vi "Main.vi"(8 "error in":errorcluster, 11 "sequenceManagerTest in":refnum<class "sequenceManagerTest.lvclass">) -> (0 "error out":errorcluster, 3 "sequenceManagerTest out":refnum<class "sequenceManagerTest.lvclass">)   [LabVIEW 2023, in "sequenceManagerTest.lvclass"]
doc: "The <b>Queued Message Handler</b> of the Worker that owns this VI."
uses:
  sequenceManagerTest.lvclass
  sequenceManagerTest.lvclass/sequenceManagerTest.ctl
  Initialization Data.ctl
  Response Cases.ctl
  <vilib>/addons/_Workers/Library/Classes/Message Queue/Message Queue.lvclass
  sequenceManagerWorker/sequenceManagerWorker.lvclass
  sequenceManagerWorker/ZE_Easy.Sequencer.lvlibp/Step/Step.lvclass
panel:
  in  "Close Button":bool
  out "Name":string
  out "IsSynchronous":bool
  out "IsParallel":bool
  out "Documentation":string
  in  "Forward Button":bool
  in  "Open Manager":bool
  in  "Path to JSON sequence file":path
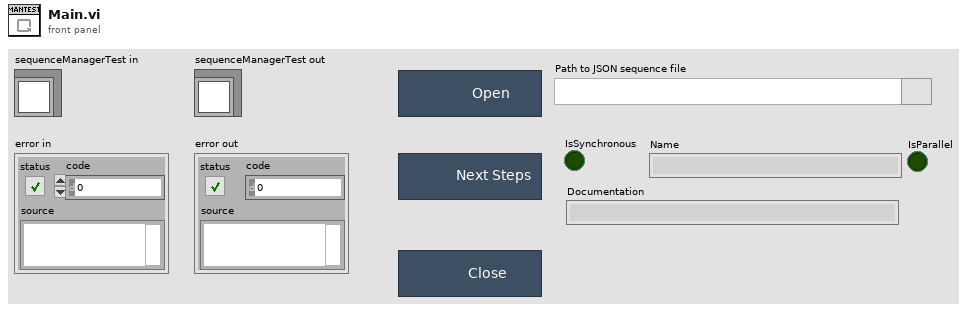
[diagram p1: front panel]
types:
  T1 = typedef "sequenceManagerTest.lvclass/Initialization Data.ctl" = cluster{"Response Cases":T2}
  T2 = typedef "sequenceManagerTest.lvclass/Response Cases.ctl" = cluster{"Placeholder - Can be deleted":string}
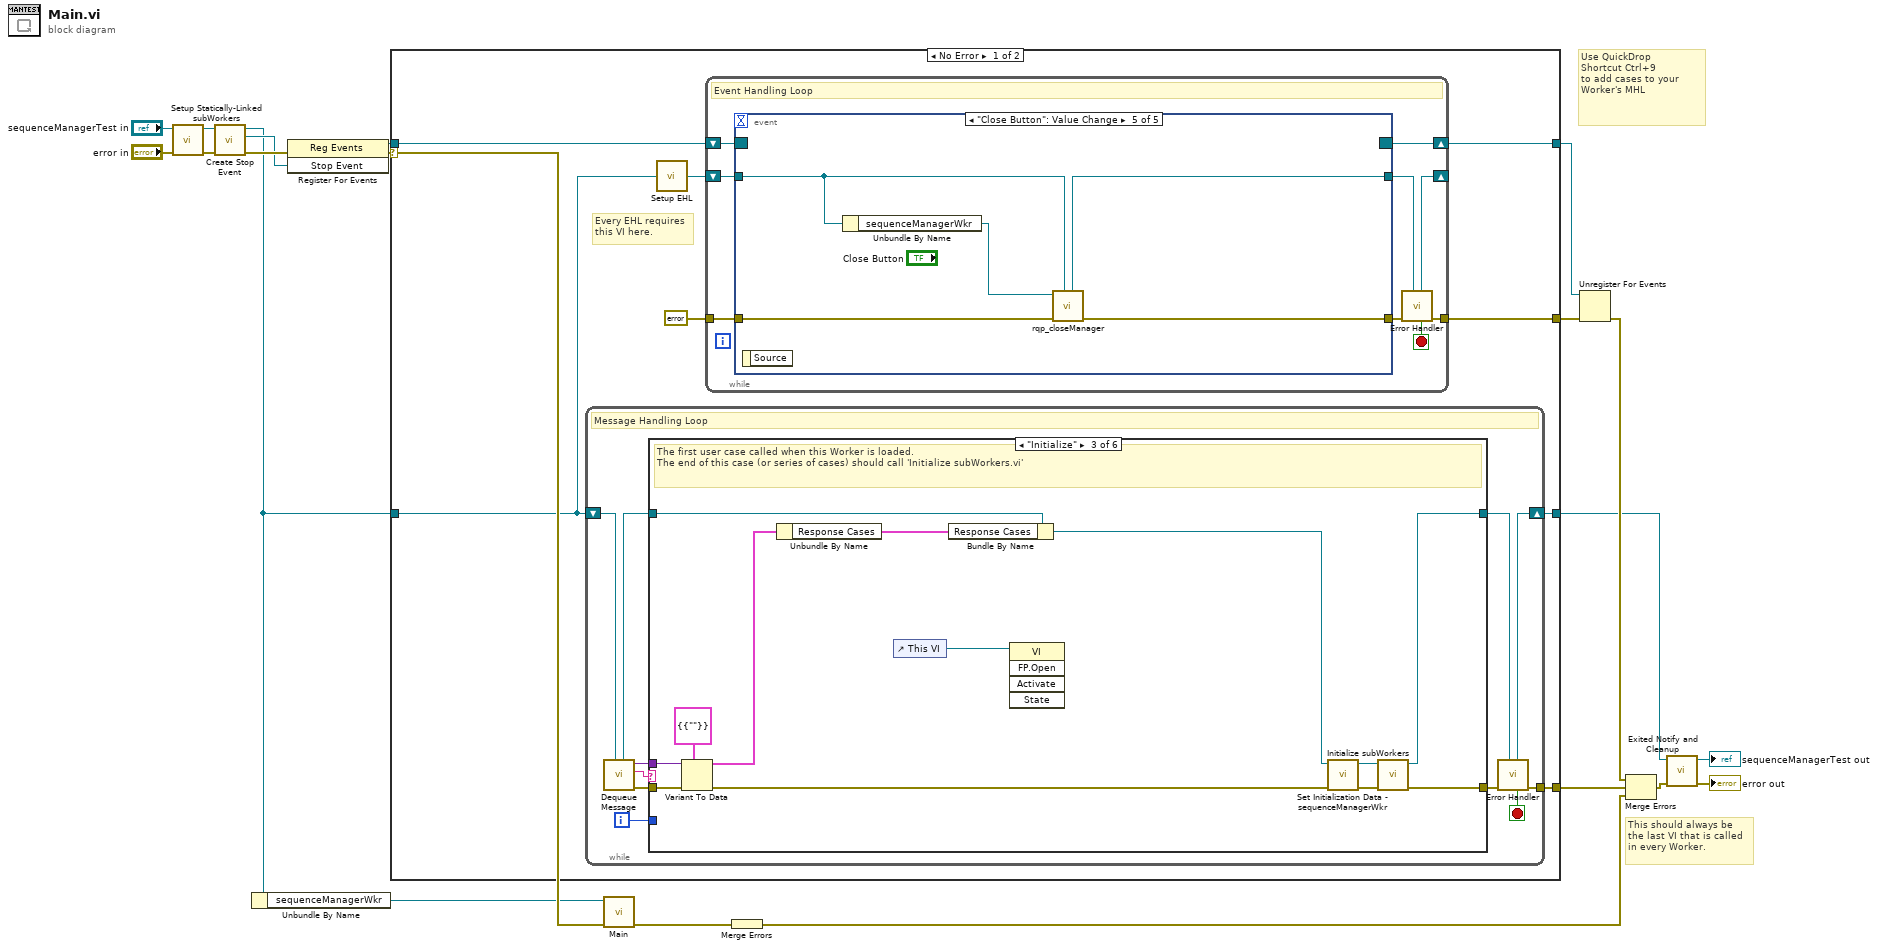
[diagram p0: block diagram]
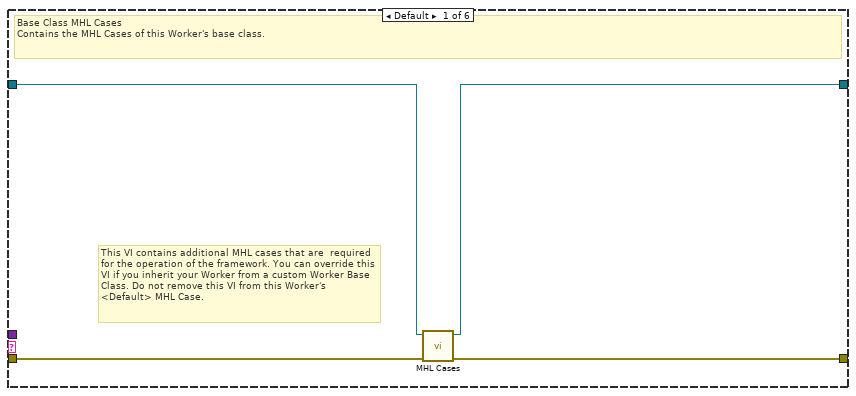
[diagram p2: hidden frame]
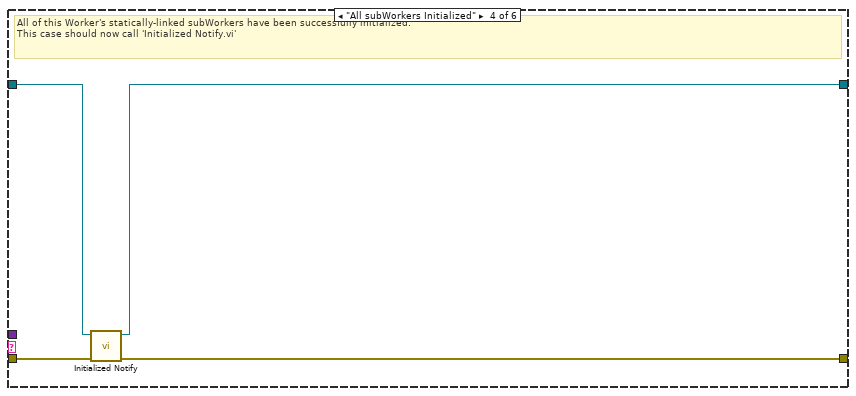
[diagram p4: hidden frame]
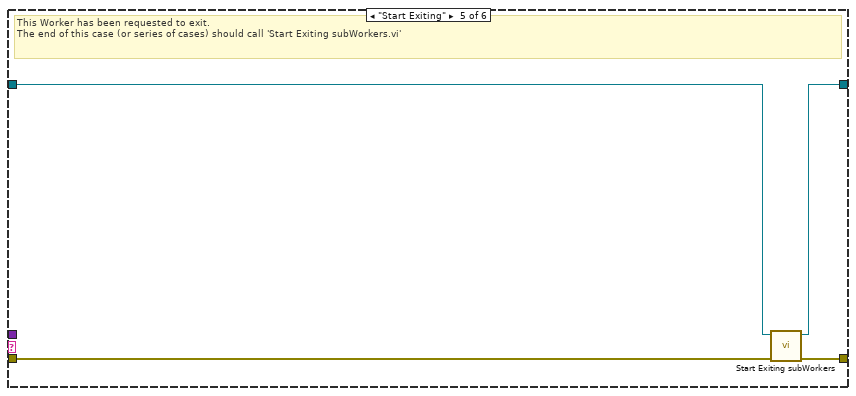
[diagram p5: hidden frame]
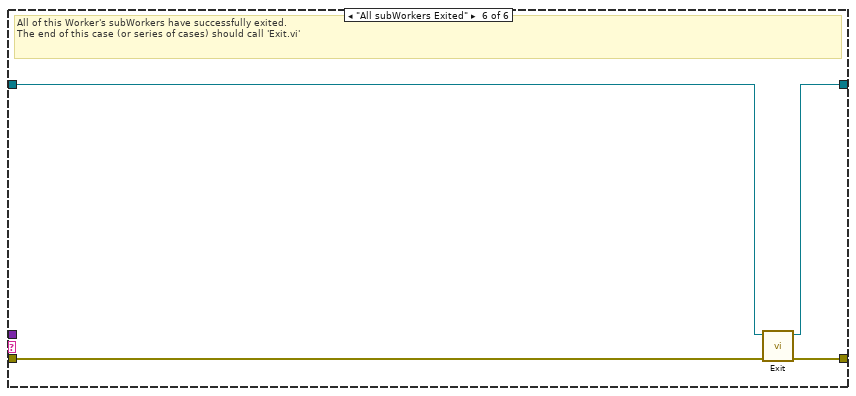
[diagram p6: hidden frame]
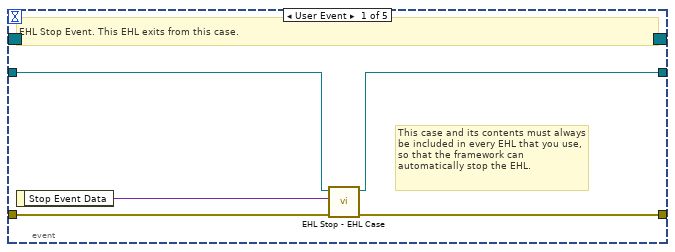
[diagram p7: hidden frame]
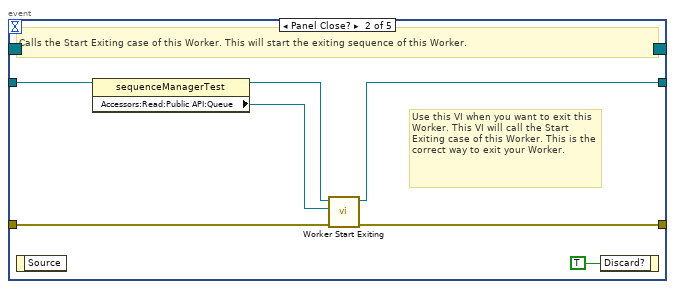
[diagram p8: hidden frame]
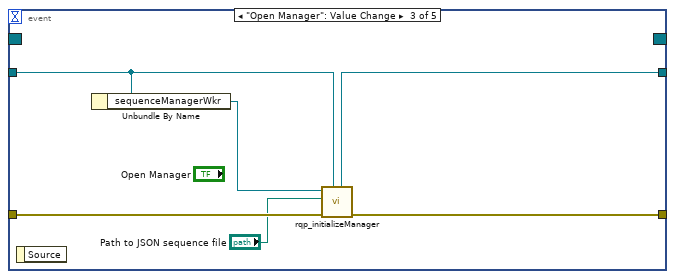
[diagram p9: hidden frame]
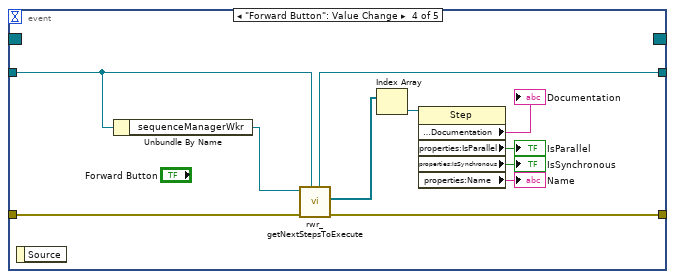
[diagram p10: hidden frame]
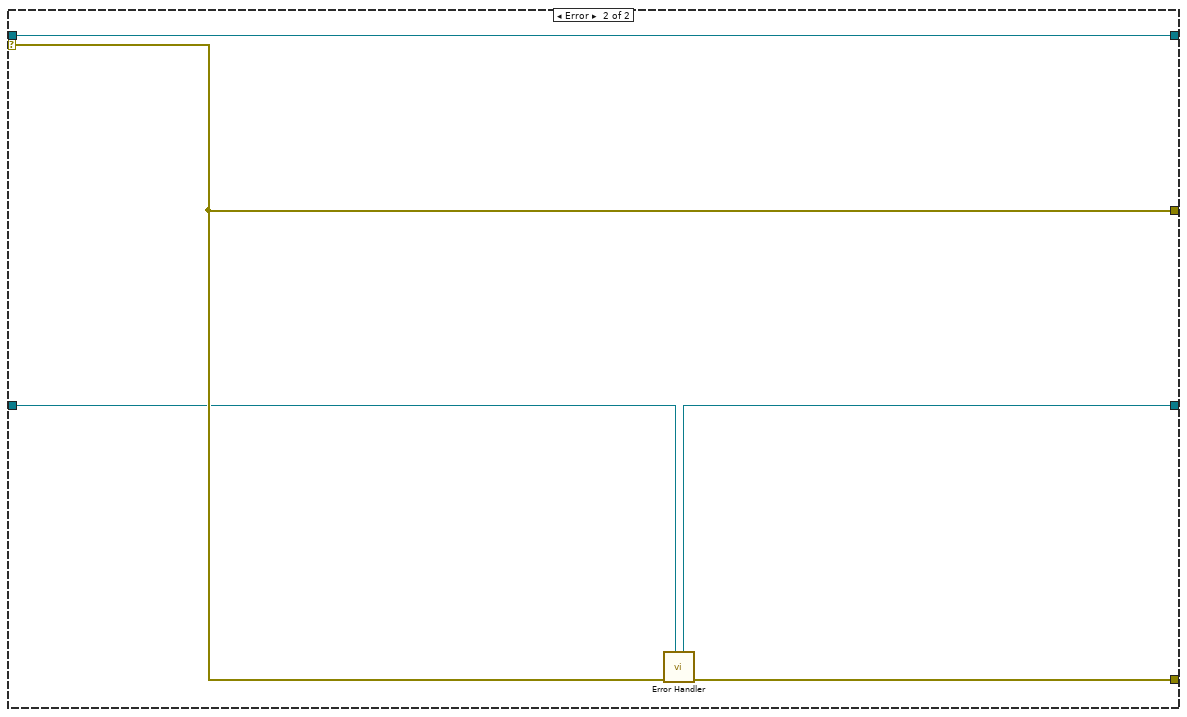
[diagram p11: hidden frame]
diagram:
  # "Use QuickDrop\nShortcut Ctrl+9\nto add cases to your\nWorker's MHL"
  # "This should always be the last VI that is called in every Worker."
  n1 = call "Setup Statically-Linked subWorkers.vi"("error in"="error in", "sequenceManagerTest in"="sequenceManagerTest in") -> ("error out"=w6:errorcluster, "sequenceManagerTest out"=w4:refnum<class "sequenceManagerTest.lvclass">)  [unwired: 8 in]
  n2 = call-dynamic "Create Stop Event.vi"("error in"=w6, "Worker"=w4) -> ("error out"=w15:errorcluster, "Stop Event"=w12:refnum<user-event>, "Worker out"=w9:refnum<class "sequenceManagerTest.lvclass">)  [unwired: 7 in]
  n3 = Unbundle By Name(w9) -> ("sequenceManagerWkr"=w1:refnum<class "sequenceManagerWorker.lvclass">)
  n4 = register-events(error in=w15, w12) -> (reference out=w14:refnum<event-registration>, error out=w7:errorcluster)  [unwired: 1 in]
  n5 = case shown="No Error" w7 {
    tunnel: w9 -> [w23 w115]
    tunnel: [w21 w116] -> w13
    tunnel: w14 -> [w28 w117]
    tunnel: [w25 w118] -> w19
    tunnel: [w27 w117] -> w18
    tunnel: [w22 w114] -> w16
    selector: w7 -> [_ w118]
    frame No Error {
      # "Every EHL requires\nthis VI here."
      n6 = while {
        shift-right: [w37] -> w22
        shift-left: w23 -> [w39]
        tunnel: [w38] -> w21
        i -> [w29]
        stop <- w30 stop-if-true
        # "Message Handling Loop"
        n7 = call-dynamic "Dequeue Message.vi"("Worker"=w39) -> ("error out"=w36:errorcluster, "Case out"=w31:string, "Data out"=w32:variant, "Worker out"=w34:refnum<class "sequenceManagerTest.lvclass">)  [unwired: 6 in, 1 out]
        n8 = case "Worker MHL Case Structure (DO NOT CHANGE LABEL NAME)" shown="\"Initialize\"" w31 {
          tunnel: w36 -> [w43 w44 w56 w60 w63 w70]
          tunnel: [w42 w44 w58 w59 w66 w69] -> w35
          tunnel: w34 -> [w41 w45 w55 w62 w64 w68]
          tunnel: [w40 w45 w57 w61 w65 w67] -> w33
          tunnel: w32 -> [_ _ w53 _ _ _]
          tunnel: w29 -> [_ _ _ _ _ _]
          frame Default {
            # "This VI contains additional MHL cases that are  required for the operation of the framework. You can override this VI if you inherit your Worker from a custom Worker Base Class. Do not remove this VI from this Worker's <Default> MHL Case."
            # "Base Class MHL Cases\nContains the MHL Cases of this Worker's base class."
            n9 = call-dynamic "MHL Cases.vi"("error in"=w43, "Worker in"=w41) -> ("error out"=w42:errorcluster, "Worker out"=w40:refnum<class "sequenceManagerTest.lvclass">)  [unwired: 8 in]
          }
          frame "------------ FRAMEWORK CASES -----------" {
            # "Start of Workers Framework Cases"
          }
          frame "Initialize" {
            # "The first user case called when this Worker is loaded.\nThe end of this case (or series of cases) should call 'Initialize subWorkers.vi'"
            n10 = Variant To Data(error in=w56, type=T1 {"Response Cases"={"Placeholder - Can be deleted"=""}} ("Initialization Data"), Variant=w53) -> (data=w52:T1, error out=w54:errorcluster)
            n11 = Unbundle By Name(w52) -> ("Response Cases"=w51:T2)
            n12 = control-ref of="This VI"() -> (w46:refnum<vi>)
            n13 = Bundle By Name(cluster=w55, "Response Cases"=w51) -> (w47:refnum<class "sequenceManagerTest.lvclass">)
            n14 = invoke class="VI" method="FP.Open"(reference=w46) -> ()  [unwired: 4 in, 5 out]
            n15 = call "Set Initialization Data - sequenceManagerWkr.vi"("error in"=w54, "sequenceManagerTest in"=w47) -> ("error out"=w49:errorcluster, "sequenceManagerTest out"=w48:refnum<class "sequenceManagerTest.lvclass">)  [unwired: 8 in]
            n16 = call-dynamic "Initialize subWorkers.vi"("error in"=w49, "Worker"=w48) -> ("error out"=w58:errorcluster, "dup Worker out"=w57:refnum<class "sequenceManagerTest.lvclass">)  [unwired: 8 in]
          }
          frame "All subWorkers Initialized" {
            # "All of this Worker's statically-linked subWorkers have been successfully initialized.\nThis case should now call 'Initialized Notify.vi'"
            n17 = call-dynamic "Initialized Notify.vi"("error in"=w60, "Worker"=w62) -> ("error out"=w59:errorcluster, "dup Worker out"=w61:refnum<class "sequenceManagerTest.lvclass">)  [unwired: 8 in]
          }
          frame "Start Exiting" {
            # "This Worker has been requested to exit. \nThe end of this case (or series of cases) should call 'Start Exiting subWorkers.vi'"
            n18 = call-dynamic "Start Exiting subWorkers.vi"("error_in"=w63, "Worker"=w64) -> ("error out"=w66:errorcluster, "dup Worker out"=w65:refnum<class "sequenceManagerTest.lvclass">)  [unwired: 8 in]
          }
          frame "All subWorkers Exited" {
            # "All of this Worker's subWorkers have successfully exited. \nThe end of this case (or series of cases) should call 'Exit.vi'"
            n19 = call-dynamic "Exit.vi"("error_in"=w70, "Worker"=w68) -> ("error out"=w69:errorcluster, "dup Worker out"=w67:refnum<class "sequenceManagerTest.lvclass">)  [unwired: 8 in]
          }
        }
        n20 = call-dynamic "Error Handler.vi"("Worker"=w33, "error_in"=w35) -> ("error out"=w38:errorcluster, "Stop Loop"=w30:bool, "Worker out"=w37:refnum<class "sequenceManagerTest.lvclass">)  [unwired: 7 in]
      }
      n21 = call-dynamic "Setup EHL.vi"("Worker"=w23) -> ("Worker out"=w24:refnum<class "sequenceManagerTest.lvclass">)  [unwired: 14 in]
      n22 = while "Event Handling Loop" {
        shift-right: [w79] -> w27
        shift-left: w28 -> [w78]
        tunnel: [w74] -> w25
        tunnel: errorcluster {"status"=FALSE, "code"=0, "source"=""} ("error constant") -> [w76]
        shift-right: [w72] -> _
        shift-left: w24 -> [w77]
        stop <- w71 stop-if-true
        # "Event Handling Loop"
        n23 = event shown="[4] \"Close Button\": Value Change" {
          selector: w78 -> [_ _ _ _ _]
          dyn-events: [_ _ _ _ _] -> w79
          timeout: _ -> [_ _ _ _ _]
          tunnel: [w83 w90 w97 w108 w113] -> w75
          tunnel: w76 -> [w84 w89 w96 w107 w112]
          tunnel: w77 -> [w82 w88 w93 w104 w109]
          tunnel: [w81 w87 w94 w105 w110] -> w73
          event User Event {
            # "This case and its contents must always be included in every EHL that you use, so that the framework can automatically stop the EHL."
            # "EHL Stop Event. This EHL exits from this case."
            n24 = event-data() -> ("Stop Event Data"=w80:variant)  [unwired: 1 in]
            n25 = call-dynamic "EHL Stop - EHL Case.vi"("error in"=w84, "Stop Event Data"=w80, "Worker"=w82) -> ("error out"=w83:errorcluster, "Worker out"=w81:refnum<class "sequenceManagerTest.lvclass">)  [unwired: 7 in]
          }
          event Panel Close? {
            # "Use this VI when you want to exit this Worker. This VI will call the Start Exiting case of this Worker. This is the correct way to exit your Worker."
            # "Calls the Start Exiting case of this Worker. This will start the exiting sequence of this Worker."
            n26 = event-data() -> ()  [unwired: 1 in, 1 out]
            n27 = property class="sequenceManagerTest"(reference=w88) -> (reference out=w86:refnum<class "sequenceManagerTest.lvclass">, "Accessors:Read:Public API:Queue"=w85:refnum<class "Message Queue.lvclass">)  [unwired: 1 in, 1 out]
            n28 = call-dynamic "Worker Start Exiting.vi"("error_in"=w89, "Message Queue"=w85, "Worker"=w86) -> ("error out"=w90:errorcluster, "dup Worker out"=w87:refnum<class "sequenceManagerTest.lvclass">)  [unwired: 7 in]
            n29 = event-data ("Event Filter Node")("Discard?"=TRUE) -> ()  [unwired: 1 in, 1 out]
          }
          event "Open Manager": Value Change {
            n30 = event-data() -> ()  [unwired: 1 in, 1 out]
            n31 = Unbundle By Name(w93) -> ("sequenceManagerWkr"=w95:refnum<class "sequenceManagerWorker.lvclass">)
            n32 = call "rqp_initializeManager.vi"("Caller in"=w93, "error in"=w96, "Path to JSON sequence file"="Path to JSON sequence file", "sequenceManagerWorker in"=w95) -> ("error out"=w97:errorcluster, "dup Caller out"=w94:refnum<class "sequenceManagerTest.lvclass">)  [unwired: 5 in, 1 out]
          }
          event "Forward Button": Value Change {
            n33 = event-data() -> ()  [unwired: 1 in, 1 out]
            n34 = Unbundle By Name(w104) -> ("sequenceManagerWkr"=w106:refnum<class "sequenceManagerWorker.lvclass">)
            n35 = call "rwr_getNextStepsToExecute.vi"("Caller in"=w104, "error in"=w107, "sequenceManagerWorker in"=w106) -> ("error out"=w108:errorcluster, "StepsToExecuteInParallel"=w103:refnum<class "Step.lvclass">[], "dup Caller out"=w105:refnum<class "sequenceManagerTest.lvclass">)  [unwired: 5 in, 1 out]
            n36 = Index Array(array=w103) -> (element=w102:refnum<class "Step.lvclass">)  [unwired: 1 in]
            n37 = property class="Step"(reference=w102) -> ("properties:Documentation"=→"Documentation":string, "properties:IsParallel"=→"IsParallel":bool, "properties:IsSynchronous"=→"IsSynchronous":bool, "properties:Name"=→"Name":string)  [unwired: 1 in, 2 out]
          }
          event "Close Button": Value Change {
            n38 = event-data() -> ()  [unwired: 1 in, 1 out]
            n39 = Unbundle By Name(w109) -> ("sequenceManagerWkr"=w111:refnum<class "sequenceManagerWorker.lvclass">)
            n40 = call "rqp_closeManager.vi"("Caller in"=w109, "error in"=w112, "sequenceManagerWorker in"=w111) -> ("error out"=w113:errorcluster, "dup Caller out"=w110:refnum<class "sequenceManagerTest.lvclass">)  [unwired: 6 in, 1 out]
          }
        }
        n41 = call-dynamic "Error Handler.vi"("Worker"=w73, "error_in"=w75) -> ("error out"=w74:errorcluster, "Stop Loop"=w71:bool, "Worker out"=w72:refnum<class "sequenceManagerTest.lvclass">)  [unwired: 7 in]
      }
    }
    frame Error {
      n42 = call-dynamic "Error Handler.vi"("Worker"=w115, "error_in"=w118) -> ("error out"=w116:errorcluster, "Worker out"=w114:refnum<class "sequenceManagerTest.lvclass">)  [unwired: 7 in, 1 out]
    }
  }
  n43 = call-dynamic "Main.vi"("error in"=w7, "sequenceManagerWorker in"=w1) -> ("error out"=w3:errorcluster)  [unwired: 8 in, 1 out]
  n44 = Merge Errors(w3) -> (w2:errorcluster)
  n45 = Unregister For Events(event registration refnum=w18, error in=w19) -> (error out=w20:errorcluster)
  n46 = Merge Errors(w20, w13, w2) -> (w17:errorcluster)
  n47 = call-dynamic "Exited Notify and Cleanup.vi"("error_in"=w17, "Worker"=w16) -> ("error out"=→"error out":errorcluster, "dup Worker out"=→"sequenceManagerTest out":refnum<class "sequenceManagerTest.lvclass">)  [unwired: 8 in]
